vi "Configure Schedule.vi"(0 "VISA resource name":refnum<visa-resource-name>, 1 "Schedule Number (1)":i32=1 min=1 max=12 step=1, 2 "Enable Schedule (Off)":bool, 3 "Due Date":T1={"Month (Jan)"=1, "Day (1)"=1, "Year (2016)"=2016} {"Year (2016)" min=2001 max=2035; "Day (1)" min=1 max=31; "Month (Jan)" items=["Jan"=1, "Feb"=2, "Mar"=3, "Apr"=4, "May"=5, "Jun"=6, "Jul"=7, "Aug"=8, "Sep"=9, "Oct"=10, "Nov"=11, "Dec"=12]}, 4 "Daily Reminder (5: 5days before)":u16(ring)=5 items=["1day before"=1, "2days before"=2, "3days before"=3, "4days before"=4, "5days before"=5, "6days before"=6, "7days before"=7, "8days before"=8, "9days before"=9, "10days before"=10], 5 "Re-notification Cycle (2: 1h)":u16(ring)=2 items=["10min", "30min", "1h", "8h", "24h"], 7 "error in (no error)":errorcluster, 9 "Buzzer (Off)":bool, 11 "Cariburation Correction (Off)":bool) -> (20 "VISA resource name out":refnum<visa-resource-name>, 27 "error out":errorcluster)   [LabVIEW 2020, in "Yokogawa GX Series.lvlib"]
doc: "Sets caliburation reminder.\n\nCommand: SSchedule"
uses:
  <instrlib>/Yokogawa GX Series/Yokogawa GX Series.lvlib
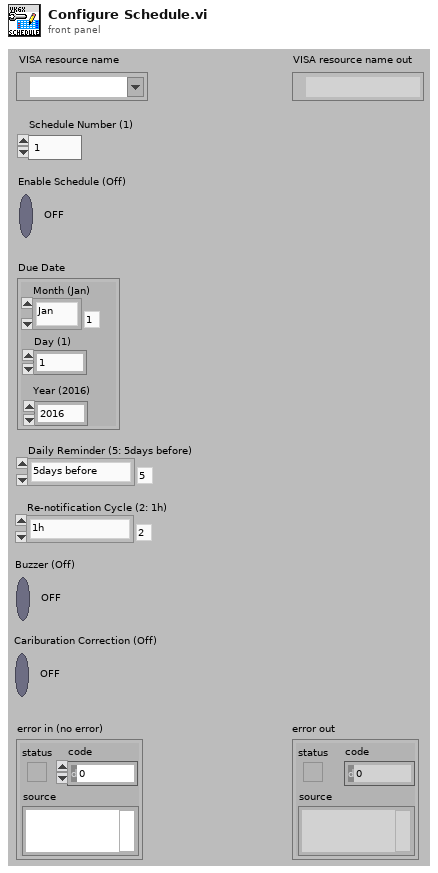
[diagram p1: front panel]
types:
  T1 = cluster{"Month (Jan)":u16, "Day (1)":i32, "Year (2016)":i32}
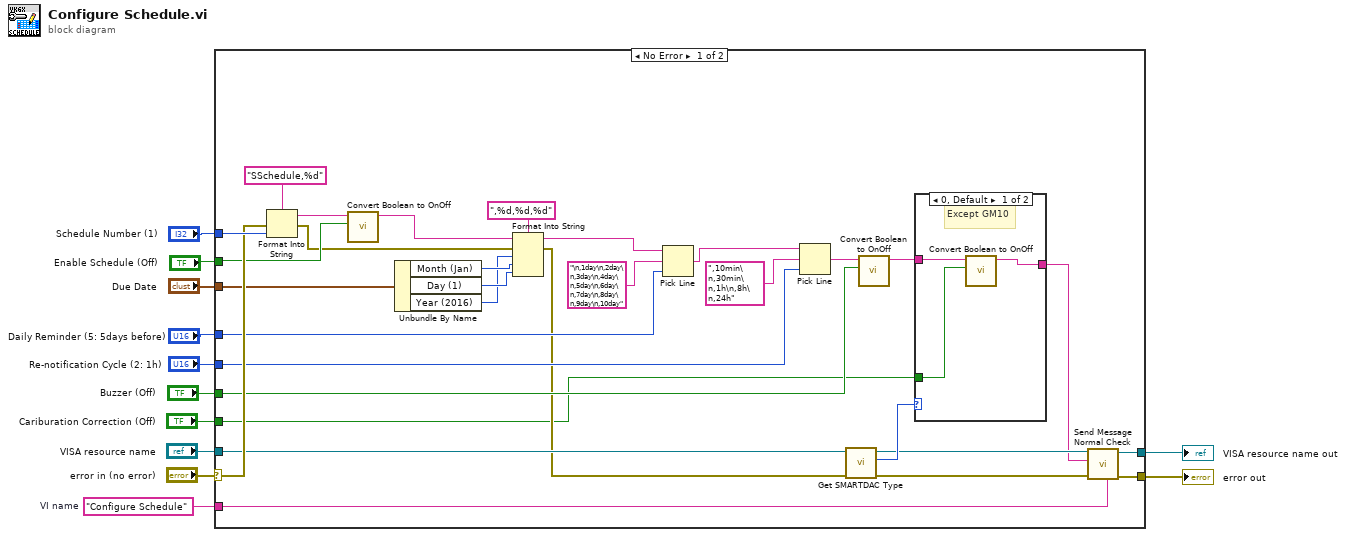
[diagram p0: block diagram]
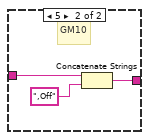
[diagram p2: hidden frame]
diagram:
  w8 = "Configure Schedule"  # VI name
  n1 = case shown="No Error" "error in (no error)" {
    selector: "error in (no error)" -> [w37 w50]
    tunnel: "VISA resource name" -> [w19 w51]
    tunnel: "Daily Reminder (5: 5days before)" -> [w25 _]
    tunnel: [w43 w51] -> w10
    tunnel: [w42 w50] -> w9
    tunnel: w8 -> [w41 _]
    tunnel: "Enable Schedule (Off)" -> [w35 _]
    tunnel: "Schedule Number (1)" -> [w38 _]
    tunnel: "Due Date" -> [w34 _]
    tunnel: "Re-notification Cycle (2: 1h)" -> [w23 _]
    tunnel: "Buzzer (Off)" -> [w20 _]
    tunnel: "Cariburation Correction (Off)" -> [w16 _]
    frame No Error {
      n2 = Format Into String(format string="SSchedule,%d", error in=w37, w38) -> (resulting string=w36:string, error out=w32:errorcluster)  [unwired: 1 in]
      n3 = call <instrlib>:"Convert Boolean to OnOff.vi"("On/Off"=w35, "Initial String (\"\")"=w36) -> ("Resulting String"=w31:string)  [unwired: 9 in]
      n4 = Unbundle By Name(w34) -> ("Month (Jan)"=w30:u16, "Day (1)"=w29:i32, "Year (2016)"=w28:i32)
      n5 = Format Into String(format string=",%d,%d,%d", initial string=w31, error in=w32, w28, w30, w29) -> (resulting string=w26:string, error out=w18:errorcluster)
      n6 = Pick Line(string ("")=w26, multi-line string="\n,1day\n,2day\n,3day\n,4day\n,5day\n,6day\n,7day\n,8day\n,9day\n,10day", line index=w25) -> (output string=w24:string)
      n7 = Pick Line(string ("")=w24, multi-line string=",10min\n,30min\n,1h\n,8h\n,24h", line index=w23) -> (output string=w21:string)
      n8 = call <instrlib>:"Get SMARTDAC Type.vi"("error in (no error)"=w18, "VISA resource name"=w19) -> ("error out"=w14:errorcluster, "SMARTDAC+ Type"=w17:u16, "VISA resource name out"=w15:refnum<visa-resource-name>)  [unwired: 7 in]
      n9 = call <instrlib>:"Convert Boolean to OnOff.vi"("On/Off"=w20, "Initial String (\"\")"=w21) -> ("Resulting String"=w40:string)  [unwired: 9 in]
      n10 = case shown="0, Default" w17 {
        tunnel: w40 -> [w46 w49]
        tunnel: w16 -> [w45 _]
        tunnel: [w44 w47] -> w13
        frame 0, Default {
          # "Except GM10"
          n11 = call <instrlib>:"Convert Boolean to OnOff.vi"("On/Off"=w45, "Initial String (\"\")"=w46) -> ("Resulting String"=w44:string)  [unwired: 9 in]
        }
        frame 5 {
          # "GM10"
          n12 = Concatenate Strings(w49, ",Off") -> (w47:string)
        }
      }
      n13 = call <instrlib>:"Send Message Normal Check.vi"("Source (\"\")"=w41, "error in (no error)"=w14, "Send Message (\"\")"=w13, "VISA resource name"=w15) -> ("error out"=w42:errorcluster, "VISA resource name out"=w43:refnum<visa-resource-name>)  [unwired: 2 in, 4 out]
    }
    frame Error {
    }
  }
  "error out" <- w9
  "VISA resource name out" <- w10
